vi "Basic Interface.vi"() -> ()   [LabVIEW 2019]
uses:
  source code/LSL components/scripts/scripts manager/scripts manager.lvclass
  source code/LSL components/output terminal/Plain OT/PainOutputTerminal.lvclass
  D:/Pet Projects/LSL/source code/LSL components/output terminal/Base/Output Terminal.lvclass
  source code/LSL components/output terminal/Plain OT/PainOutputTerminal.lvclass/PainOutputTerminal.ctl
  source code/LSL components/variables/RT Variables/RT Variables.lvclass
  source code/LSL components/scripts/scripts manager/scripts manager.lvclass/scripts manager.ctl
  source code/LSL components/output terminal/Plain OT/properties/Write Output Terminal.vi
  source code/LSL components/scripts/scripts manager/properties/Write Scripts.vi
panel:
  in  "Help":bool
  in  "Script Compile":bool
  in  "Script Save":bool
  in  "Script Delete":bool
  in  "Script New":bool
  in  "Script Run":bool
  in  "Script Files":i32(listbox)
  out "Output Terminal":string
  in  "scripting pane":T1
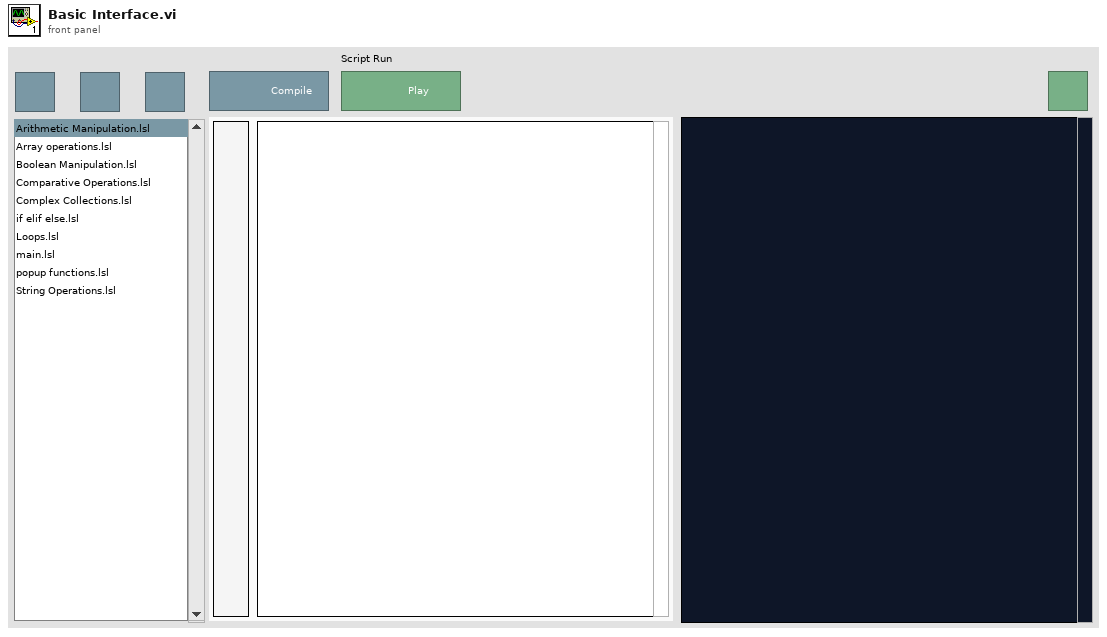
[diagram p1: front panel]
types:
  T1 = cluster{"Script Editor":string, "Script Editor":string}
  T2 = enum32{"Invalid", "Standard", "Closed", "Hidden", "Minimized", "Maximized"}
  T3 = enum32{"invalid app kind", "Development System", "Run Time System", "Student Edition", "Embedded LabVIEW", "Evaluation", "Custom"}
  T4 = cluster{"Core":cluster{"Current VI Reference":refnum<vi>, "Close Panel on Exit?":bool}, "scripts manager":refnum<class "scripts manager.lvclass">, "Script":string, "Config Folder":path, "PainOT":refnum<class "PainOutputTerminal.lvclass">}
  T5 = cluster{"Current VI Reference":refnum<vi>, "Close Panel on Exit?":bool}
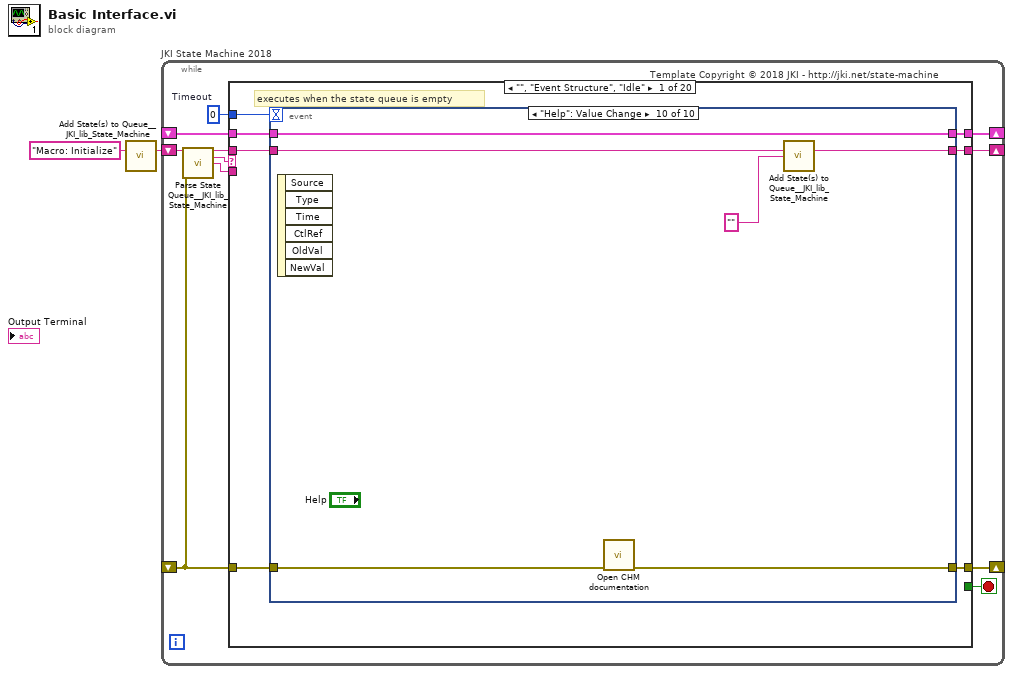
[diagram p0: block diagram]
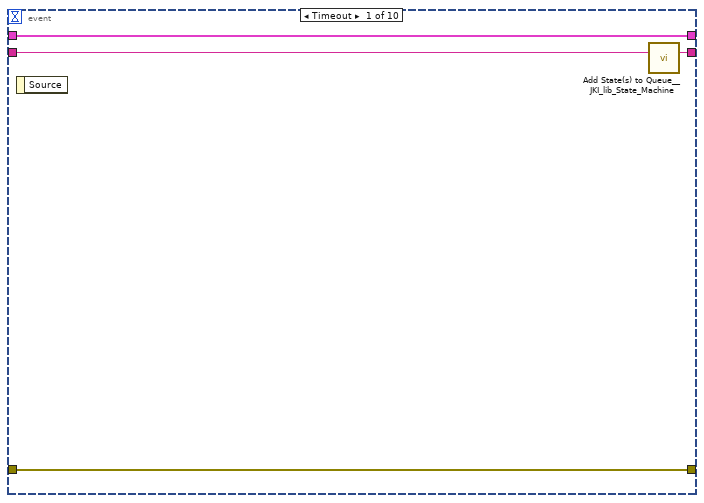
[diagram p2: hidden frame]
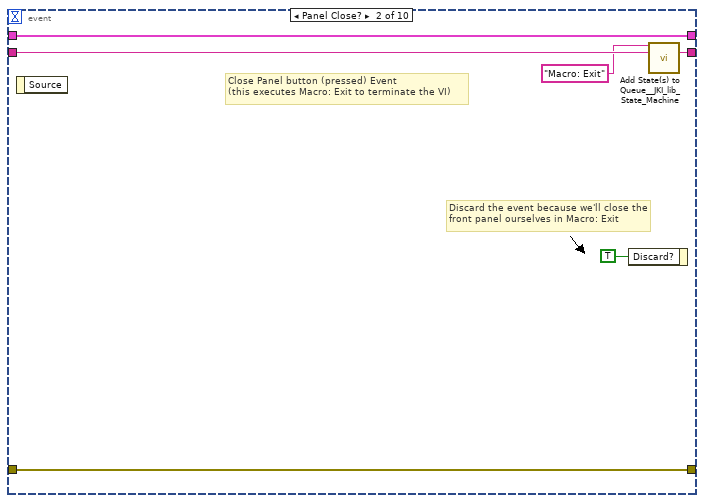
[diagram p3: hidden frame]
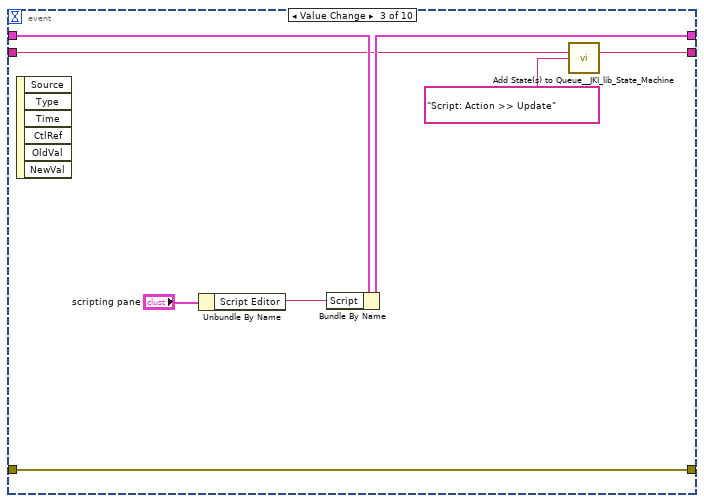
[diagram p4: hidden frame]
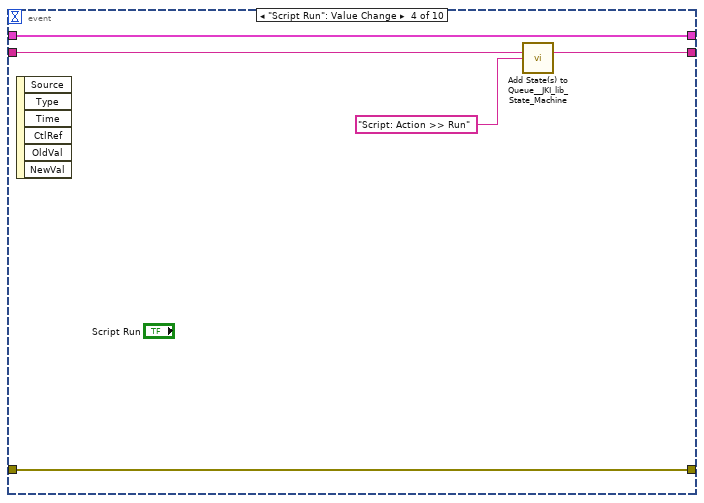
[diagram p5: hidden frame]
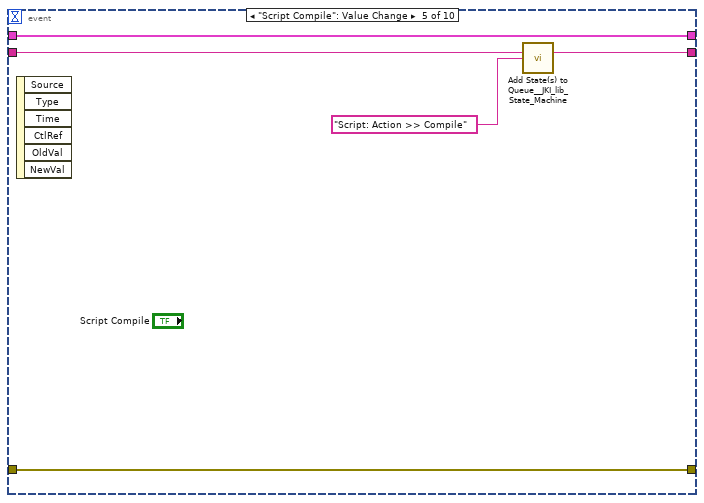
[diagram p6: hidden frame]
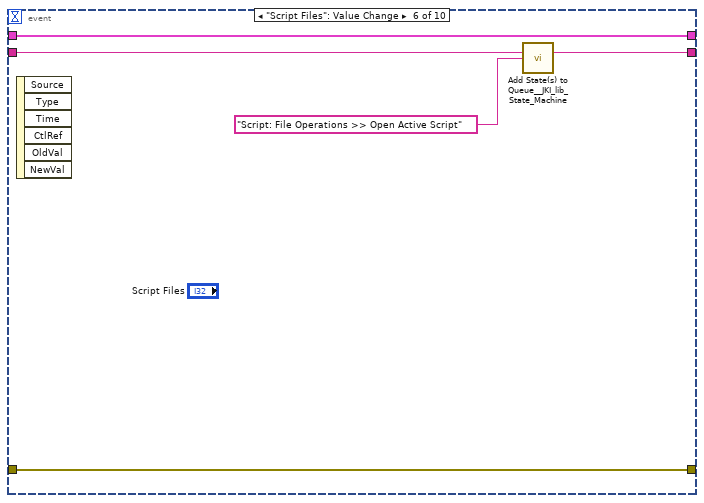
[diagram p7: hidden frame]
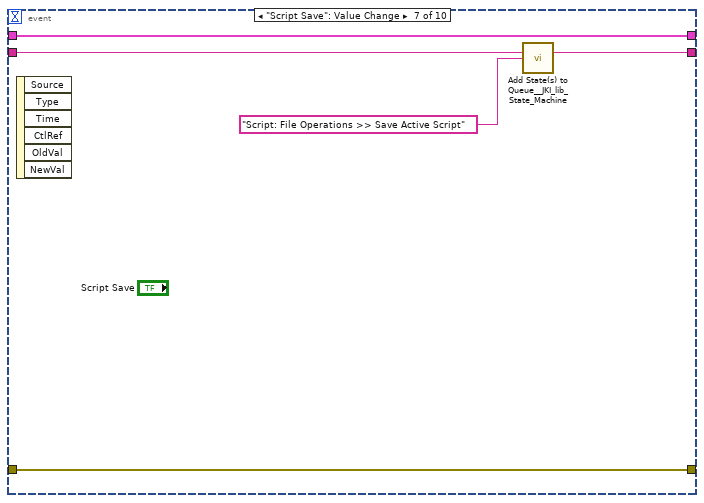
[diagram p8: hidden frame]
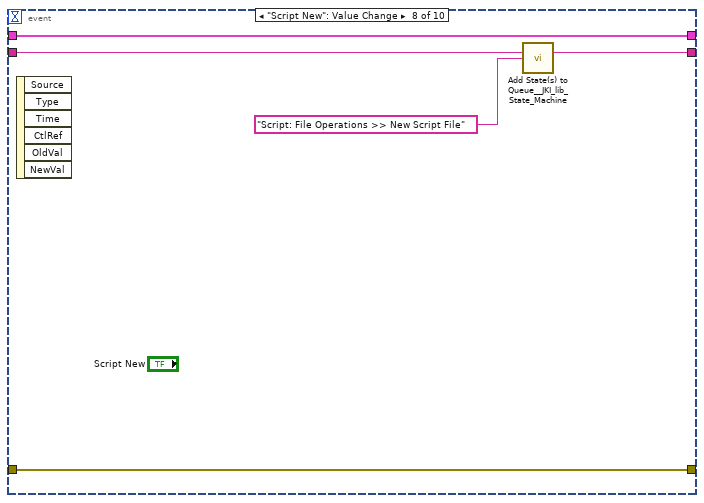
[diagram p9: hidden frame]
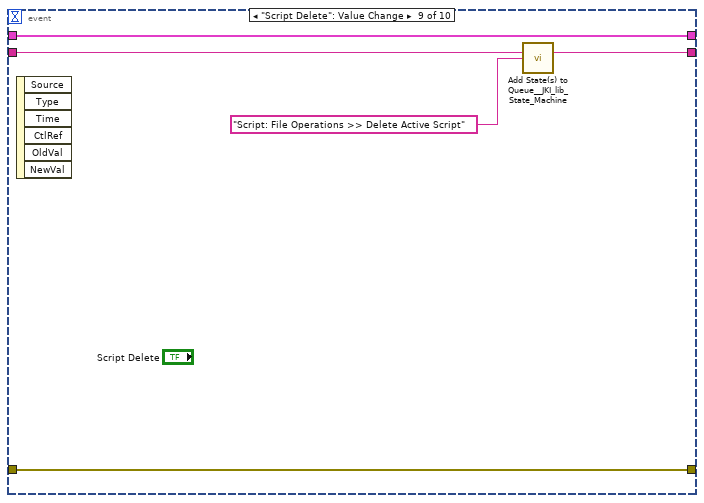
[diagram p10: hidden frame]
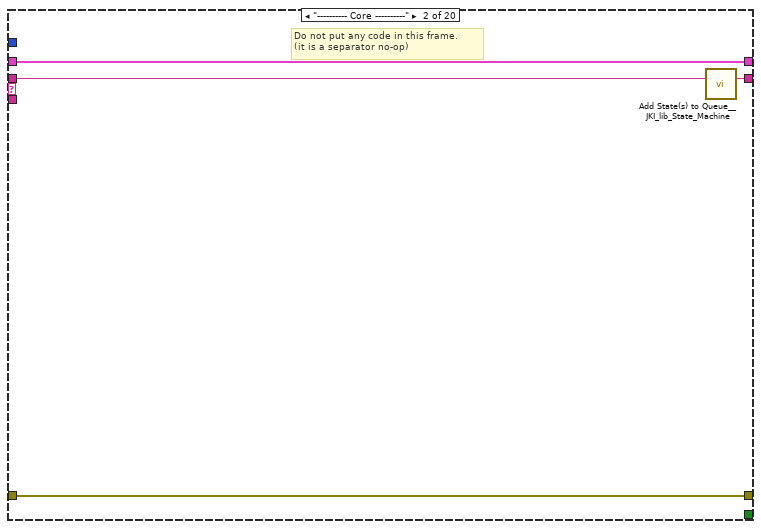
[diagram p11: hidden frame]
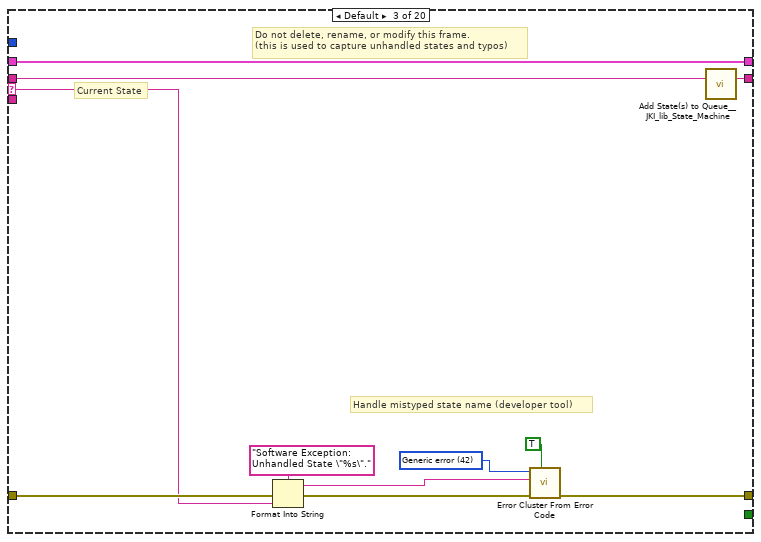
[diagram p12: hidden frame]
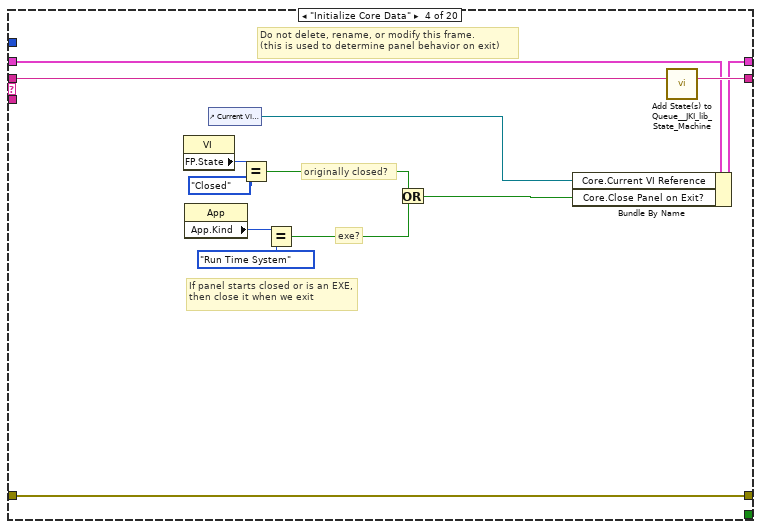
[diagram p13: hidden frame]
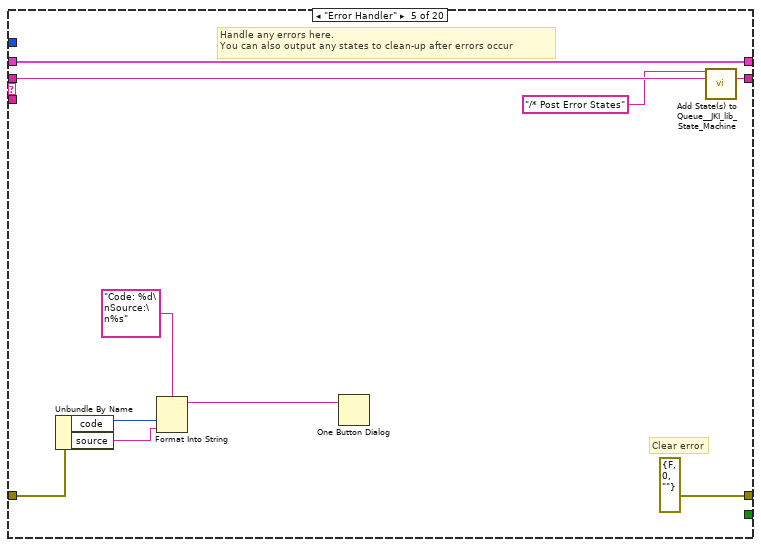
[diagram p14: hidden frame]
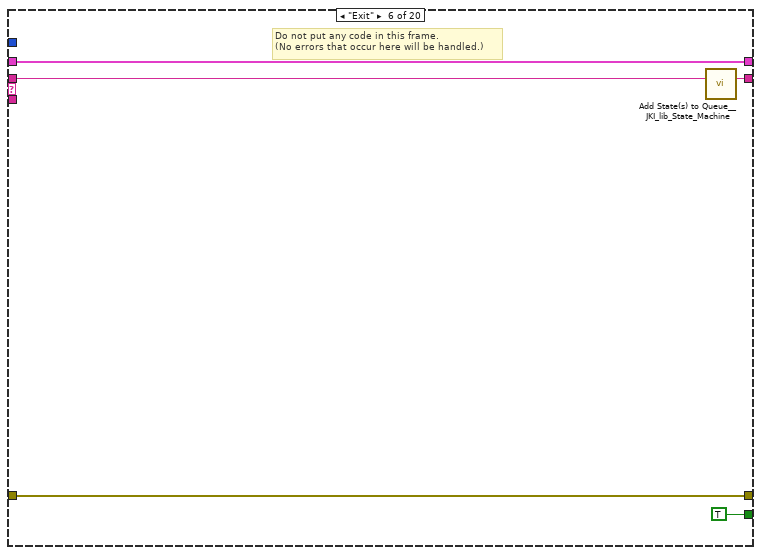
[diagram p15: hidden frame]
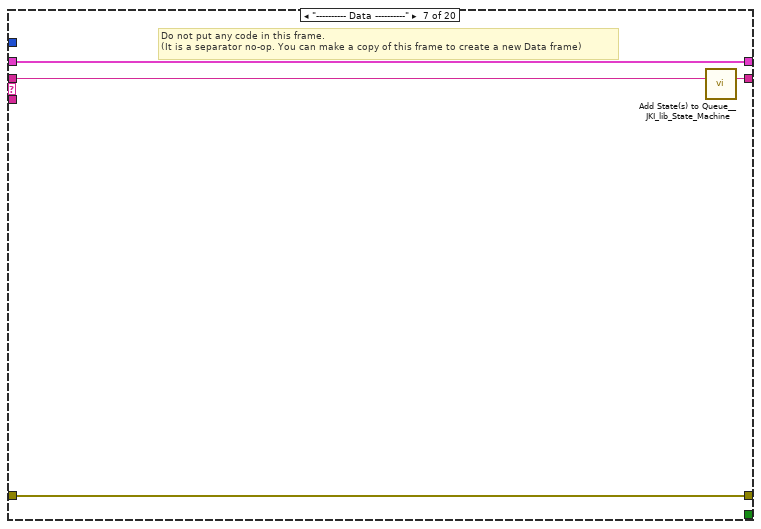
[diagram p16: hidden frame]
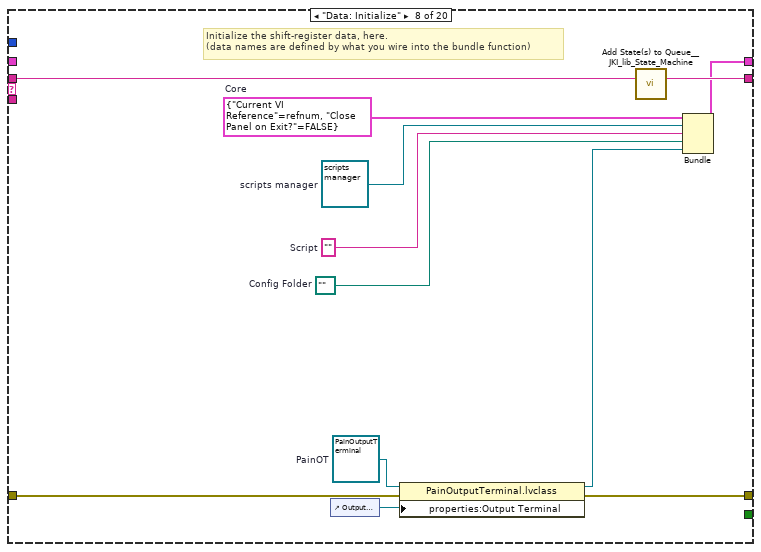
[diagram p17: hidden frame]
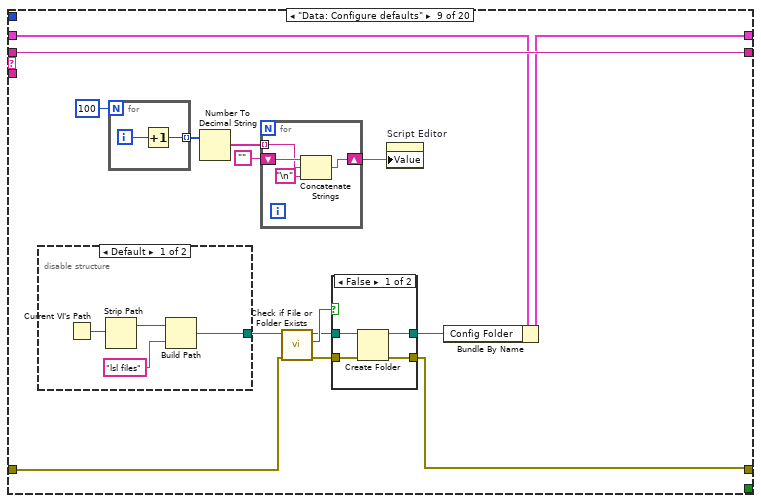
[diagram p18: hidden frame]
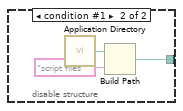
[diagram p19: hidden frame]
diagram:
  n1 = call <vilib>:"Add State(s) to Queue__JKI_lib_State_Machine.vi"("State(s) in (\"\")"="Macro: Initialize") -> ("States Out"=w2:string)  [unwired: 14 in]
  n2 = while "JKI State Machine 2018" {
    shift-right: [w6] -> _
    shift-left: _ -> [w5]
    shift-right: [w9] -> _
    shift-left: _ -> [w3]
    shift-right: [w8] -> _
    shift-left: w2 -> [w10]
    stop <- w7 stop-if-true
    w4 = 0  # Timeout
    # "Template Copyright © 2018 JKI - http://jki.net/state-machine"
    n3 = call <vilib>:"Parse State Queue__JKI_lib_State_Machine.vi"("State Queue"=w10, "Error In (no error)"=w3) -> ("Remaining States"=w12:string, "Current State"=w13:string, "Arguments"=w11:string)  [unwired: 11 in]
    n4 = case shown="\"\", \"Event Structure\", \"Idle\"" w13 {
      selector: w13 -> [_ _ w79 _ _ _ _ _ _ _ _ _ _ _ _ _ _ _ _ _]
      tunnel: w12 -> [w20 w78 w83 w102 w112 w117 w121 w133 w148 w173 w177 w189 w195 w206 w275 w280 w290 w294 w305 w335]
      tunnel: w11 -> [_ _ _ _ _ _ _ _ _ _ _ _ w190 w200 _ _ _ _ w303 w343]
      tunnel: w5 -> [w18 w75 w81 w95 w109 w115 w118 _ w141 w168 w174 w187 w193 w202 w272 w277 w287 w291 w298 w342]
      tunnel: [w17 w76 w85 w99 errorcluster {"status"=FALSE, "code"=0, "source"=""} ("error out") w114 w119 w124 w143 w169 w175 w184 w191 w203 w273 w278 w288 w292 w301 w344] -> w9
      tunnel: w3 -> [w16 w76 w84 w99 w107 w114 w119 w125 w144 w170 w175 w185 w192 w204 w273 w278 w288 w292 w302 w339]
      tunnel: [w19 w77 w82 w101 w111 w116 w120 w132 w148 w172 w176 w188 w194 w205 w274 w279 w289 w293 w304 w336] -> w8
      tunnel: [_ _ _ _ _ TRUE _ _ _ _ _ _ _ _ _ _ _ _ _ _] -> w7
      tunnel: [w15 w75 w81 w100 w109 w115 w118 w130 w140 w168 w174 w187 w193 w202 w272 w277 w287 w291 w297 w342] -> w6
      tunnel: w4 -> [w14 _ _ _ _ _ _ _ _ _ _ _ _ _ _ _ _ _ _ _]
      frame "", "Event Structure", "Idle" {
        # "executes when the state queue is empty"
        n5 = event shown="[9] \"Help\": Value Change" {
          selector: _ -> [_ _ _ _ _ _ _ _ _ _]
          dyn-events: _ -> [_ _ _ _ _ _ _ _ _ _]
          timeout: w14 -> [_ _ _ _ _ _ _ _ _ _]
          tunnel: w20 -> [w24 w30 w33 w40 w45 w50 w55 w60 w65 w72]
          tunnel: [w23 w29 w34 w41 w46 w51 w56 w61 w66 w73] -> w19
          tunnel: w18 -> [w21 w27 w36 w43 w48 w53 w58 w63 w68 w74]
          tunnel: [w22 w28 w31 w42 w47 w52 w57 w62 w67 w69] -> w17
          tunnel: w16 -> [w22 w28 w31 w42 w47 w52 w57 w62 w67 w70]
          tunnel: [w21 w27 w35 w43 w48 w53 w58 w63 w68 w74] -> w15
          event Timeout {
            n6 = event-data() -> ()  [unwired: 1 in, 1 out]
            n7 = call <vilib>:"Add State(s) to Queue__JKI_lib_State_Machine.vi"("State(s) in (\"\")"=w24) -> ("States Out"=w23:string)  [unwired: 14 in]
          }
          event Panel Close? {
            # "Discard the event because we'll close the front panel ourselves in Macro: Exit"
            # "Close Panel button (pressed) Event\n(this executes Macro: Exit to terminate the VI)"
            n8 = event-data() -> ()  [unwired: 1 in, 1 out]
            n9 = event-data("Discard?"=TRUE) -> ()  [unwired: 1 in, 1 out]
            n10 = call <vilib>:"Add State(s) to Queue__JKI_lib_State_Machine.vi"("State(s) in Front (\"\")"="Macro: Exit", "State(s) in (\"\")"=w30) -> ("States Out"=w29:string)  [unwired: 13 in]
          }
          event "scripting pane.Script Editor": Value Change {
            n11 = event-data() -> ()  [unwired: 1 in, 6 out]
            n12 = Unbundle By Name("scripting pane") -> ("Script Editor"=w37:string)
            n13 = Bundle By Name(cluster=w36, "Script"=w37) -> (w35:T4)
            n14 = call <vilib>:"Add State(s) to Queue__JKI_lib_State_Machine.vi"("State(s) in (\"\")"=w33, "State(s) at Back (\"\")"="Script: Action >> Update" ("State(s) at Back (\"\")")) -> ("States Out"=w34:string)  [unwired: 13 in]
          }
          event "Script Run": Value Change {
            n15 = event-data() -> ()  [unwired: 1 in, 6 out]
            n16 = call <vilib>:"Add State(s) to Queue__JKI_lib_State_Machine.vi"("State(s) in (\"\")"=w40, "State(s) at Back (\"\")"="Script: Action >> Run" ("State(s) at Back (\"\")")) -> ("States Out"=w41:string)  [unwired: 13 in]
          }
          event "Script Compile": Value Change {
            n17 = event-data() -> ()  [unwired: 1 in, 6 out]
            n18 = call <vilib>:"Add State(s) to Queue__JKI_lib_State_Machine.vi"("State(s) in (\"\")"=w45, "State(s) at Back (\"\")"="Script: Action >> Compile" ("State(s) at Back (\"\")")) -> ("States Out"=w46:string)  [unwired: 13 in]
          }
          event "Script Files": Value Change {
            n19 = event-data() -> ()  [unwired: 1 in, 6 out]
            n20 = call <vilib>:"Add State(s) to Queue__JKI_lib_State_Machine.vi"("State(s) in (\"\")"=w50, "State(s) at Back (\"\")"="Script: File Operations >> Open Active Script" ("State(s) at Back (\"\")")) -> ("States Out"=w51:string)  [unwired: 13 in]
          }
          event "Script Save": Value Change {
            n21 = event-data() -> ()  [unwired: 1 in, 6 out]
            n22 = call <vilib>:"Add State(s) to Queue__JKI_lib_State_Machine.vi"("State(s) in (\"\")"=w55, "State(s) at Back (\"\")"="Script: File Operations >> Save Active Script" ("State(s) at Back (\"\")")) -> ("States Out"=w56:string)  [unwired: 13 in]
          }
          event "Script New": Value Change {
            n23 = event-data() -> ()  [unwired: 1 in, 6 out]
            n24 = call <vilib>:"Add State(s) to Queue__JKI_lib_State_Machine.vi"("State(s) in (\"\")"=w60, "State(s) at Back (\"\")"="Script: File Operations >> New Script File" ("State(s) at Back (\"\")")) -> ("States Out"=w61:string)  [unwired: 13 in]
          }
          event "Script Delete": Value Change {
            n25 = event-data() -> ()  [unwired: 1 in, 6 out]
            n26 = call <vilib>:"Add State(s) to Queue__JKI_lib_State_Machine.vi"("State(s) in (\"\")"=w65, "State(s) at Back (\"\")"="Script: File Operations >> Delete Active Script" ("State(s) at Back (\"\")")) -> ("States Out"=w66:string)  [unwired: 13 in]
          }
          event "Help": Value Change {
            n27 = event-data() -> ()  [unwired: 1 in, 6 out]
            n28 = call "Open CHM documentation.vi"("error in"=w70) -> ("error out"=w69:errorcluster)  [unwired: 10 in]
            n29 = call <vilib>:"Add State(s) to Queue__JKI_lib_State_Machine.vi"("State(s) in (\"\")"=w72, "State(s) at Back (\"\")"="" ("State(s) at Back (\"\")")) -> ("States Out"=w73:string)  [unwired: 13 in]
          }
        }
      }
      frame "---------- Core ----------" {
        # "Do not put any code in this frame.\n(it is a separator no-op)"
        n30 = call <vilib>:"Add State(s) to Queue__JKI_lib_State_Machine.vi"("State(s) in (\"\")"=w78) -> ("States Out"=w77:string)  [unwired: 14 in]
      }
      frame Default {
        w88 = 42 items=["No error", "Argument error", "Memory is full", "Out of zone", "End of file", "File already open", "Generic file I/O error", "File not found", "File permission error", "Disk is full", "Duplicate path", "Too many files open", "System feature not enabled", "Resource file not found", "Cannot add resource", "Resource not found", "Image not found", "Image memory error", "Pen does not exist", "Config type invalid", "Config token not found", "Config parse error", "Config memory error", "Bad external code format", "Bad external code offset", "External code not present", "Null window", "Destroy window error", "Null menu", "Print aborted", "Bad print record", "Print driver error", "Windows error during printing", "Memory error during printing", "Print dialog error", "Generic print error", "Invalid device refnum", "Device not found", "Device parameter error", "Device unit error", "Cannot open device", "Device call aborted", "Generic error", "Cancelled by user", "Object ID too low", "Object ID too high", "Object not in heap", "Unknown heap", "Unknown object (invalid DefProc)", "Unknown object (DefProc not in table)", "Message out of range", "Invalid (null) method", "Unknown message", "Manager call not supported", "Bad address", "Network operation in progress", "Network operation timed out", "Connection is busy", "Network attribute not supported", "Network error", "Address in use", "System out of memory", "Connection aborted", "Connection refused", "Not connected", "Already connected", "Connection closed", "Initialization error (interapplication manager)", "Bad occurrence", "Wait on unbound occurrence handler", "Occurrence queue overflow", "Datalog type conflict", "Unused", "Unrecognized type (interapplication manager)", "Memory corrupt", "Failed to make temporary DLL", "Old CIN version", "Drag socket not found", "Failed to load drop-object", "Failed to register OLE object", "Failed to release OLE object", "Format specifier type mismatch", "Unknown format specifier", "Too few format specifiers", "Too many format specifiers", "Scan failed", "Newer CIN version", "Error converting to variant", "Runtime menu error", "Password tampered", "Variant attribute not found", "Incompatible variant data type", "Event data is not available", "Event Store is not present", "Occurrence is not found", "Event Queue is not created", "Event info is not available", "Refnum passed is NULL", "Error retrieving Class GUID", "Error retrieving CoClass GUID", "Error retrieving TypeLib GUID.", "Bad built application magic bytes.", "Specific driver is different from the specific driver associated with the Logical Name.", "There is no session opened to the class driver.", "Max Error", "MAX - Error with config objects", "MAX - Error loading configuration", "MAX - Group not supported"]
        # "Current State"
        # "Do not delete, rename, or modify this frame.\n(this is used to capture unhandled states and typos)"
        # "Handle mistyped state name (developer tool)"
        n31 = Format Into String(format string="Software Exception: Unhandled State \"%s\"." ("message"), error in=w84, w79) -> (resulting string=w87:string, error out=w86:errorcluster)  [unwired: 1 in]
        n32 = call <vilib>:"Error Cluster From Error Code.vi"("show call chain? (False)"=TRUE, "error in (no error)"=w86, "error message (\"\")"=w87, "error code (0)"=w88) -> ("error out"=w85:errorcluster)  [unwired: 5 in]
        n33 = call <vilib>:"Add State(s) to Queue__JKI_lib_State_Machine.vi"("State(s) in (\"\")"=w83) -> ("States Out"=w82:string)  [unwired: 14 in]
      }
      frame "Initialize Core Data" {
        # "Do not delete, rename, or modify this frame.\n(this is used to determine panel behavior on exit)"
        # "originally closed?"
        # "exe?"
        # "If panel starts closed or is an EXE, then close it when we exit"
        n34 = property class="VI"() -> ("FP.State"=w92:T2)  [unwired: 2 in, 2 out]
        n35 = property class="App"() -> ("App.Kind"=w98:T3)  [unwired: 2 in, 2 out]
        n36 = control-ref of="Current VI Reference"() -> (w93:refnum<vi>)
        n37 = Equal?(x=w92, y=T2."Closed" ("Front Panel Window:State")) -> (x = y?=w90:bool)
        n38 = Equal?(x=w98, y=T3."Run Time System" ("Application:Kind")) -> (x = y?=w96:bool)
        n39 = Or(x=w90, y=w96) -> (x .or. y?=w94:bool)
        n40 = Bundle By Name(cluster=w95, "Core.Current VI Reference"=w93, "Core.Close Panel on Exit?"=w94) -> (w100:T4)
        n41 = call <vilib>:"Add State(s) to Queue__JKI_lib_State_Machine.vi"("State(s) in (\"\")"=w102) -> ("States Out"=w101:string)  [unwired: 14 in]
      }
      frame "Error Handler" {
        # "Handle any errors here.\nYou can also output any states to clean-up after errors occur"
        # "Clear error"
        n42 = Unbundle By Name(w107) -> ("code"=w106:i32, "source"=w105:string)
        n43 = Format Into String(format string="Code: %d\nSource:\n%s", w106, w105) -> (resulting string=w103:string)  [unwired: 2 in, 1 out]
        n44 = One Button Dialog(message=w103) -> ()  [unwired: 1 in, 1 out]
        n45 = call <vilib>:"Add State(s) to Queue__JKI_lib_State_Machine.vi"("State(s) in Front (\"\")"="/* Post Error States", "State(s) in (\"\")"=w112) -> ("States Out"=w111:string)  [unwired: 13 in]
      }
      frame "Exit" {
        # "Do not put any code in this frame.\n(No errors that occur here will be handled.)"
        n46 = call <vilib>:"Add State(s) to Queue__JKI_lib_State_Machine.vi"("State(s) in (\"\")"=w117) -> ("States Out"=w116:string)  [unwired: 14 in]
      }
      frame "---------- Data ----------" {
        # "Do not put any code in this frame.\n(It is a separator no-op. You can make a copy of this frame to create a new Data frame)"
        n47 = call <vilib>:"Add State(s) to Queue__JKI_lib_State_Machine.vi"("State(s) in (\"\")"=w121) -> ("States Out"=w120:string)  [unwired: 14 in]
      }
      frame "Data: Initialize" {
        w122 = path ""  # Config Folder
        w127 = refnum<class "PainOutputTerminal.lvclass"> refnum  # PainOT
        w128 = ""  # Script
        w129 = refnum<class "scripts manager.lvclass"> refnum  # scripts manager
        w131 = T5 {"Current VI Reference"=refnum, "Close Panel on Exit?"=FALSE}  # Core
        # "Initialize the shift-register data, here.\n(data names are defined by what you wire into the bundle function)"
        n48 = control-ref of="Output Terminal"() -> (w123:refnum<vi>)
        n49 = property class="PainOutputTerminal.lvclass"(reference=w127, error in=w125, "properties:Output Terminal"=w123) -> (reference out=w126:refnum<class "PainOutputTerminal.lvclass">, error out=w124:errorcluster)
        n50 = call <vilib>:"Add State(s) to Queue__JKI_lib_State_Machine.vi"("State(s) in (\"\")"=w133) -> ("States Out"=w132:string)  [unwired: 14 in]
        n51 = Bundle("Core"=w131, "scripts manager"=w129, "Script"=w128, "Config Folder"=w122, "PainOT"=w126) -> (w130:T4)  [unwired: 1 in]
      }
      frame "Data: Configure defaults" {
        n52 = disable-structure shown="Default" {
          disable-tunnel: [w149 w153] -> w134
          frame condition #0 (active) {
            n53 = Current VI's Path() -> (path=w152:path)
            n54 = Strip Path(path=w152) -> (stripped path=w151:path)  [unwired: 1 out]
            n55 = Build Path(base path=w151, name or relative path="lsl files") -> (appended path=w149:path)
          }
          frame condition #1 {
            n56 = call <vilib>:"Application Directory.vi"() -> ("Application Directory"=w154:path)
            n57 = Build Path(base path=w154, name or relative path="script files") -> (appended path=w153:path)
          }
        }
        n58 = for {
          N: 100 -> [_]
          tunnel: [w160] -> w138 mode=indexing
          i -> [w161]
          n59 = Increment(x=w161) -> (x+1=w160:i32)
        }
        n60 = Number To Decimal String(number=w138) -> (decimal integer string=w136:string[])  [unwired: 1 in]
        n61 = for {
          tunnel: w136 -> [w156] mode=indexing
          shift-right: [w159] -> w137
          shift-left: "" -> [w157]
          n62 = Concatenate Strings(w157, w156, "\n") -> (w159:string)
        }
        n63 = call <vilib>:"Check if File or Folder Exists.vi"("error in (no error)"=w144, "path"=w134) -> ("error out"=w145:errorcluster, "file or folder exists?"=w147:bool, "dup path"=w146:path)  [unwired: 7 in]
        n64 = case shown="False" w147 {
          tunnel: w145 -> [w165 w166]
          tunnel: w146 -> [w164 w167]
          tunnel: [w162 w167] -> w142
          tunnel: [w163 w166] -> w143
          frame False {
            n65 = Create Folder(path (use dialog)=w164, error in=w165) -> (created path=w162:path, error out=w163:errorcluster)  [unwired: 1 in, 1 out]
          }
          frame True {
          }
        }
        n66 = property on="Script Editor" class="Str"("Value"=w137) -> ()  [unwired: 2 in, 2 out]
        n67 = Bundle By Name(cluster=w141, "Config Folder"=w142) -> (w140:T4)
      }
      frame "Data: Cleanup" {
        # "Cleanup any data and references, here.\n(this is called automatically, by the Macro: Exit)"
        n68 = Unbundle By Name(w168) -> ("Core.Current VI Reference"=w171:refnum<vi>)
        n69 = Close Reference(reference=w171, error in (no error)=w170) -> (error out=w169:errorcluster)
        n70 = call <vilib>:"Add State(s) to Queue__JKI_lib_State_Machine.vi"("State(s) in (\"\")"=w173) -> ("States Out"=w172:string)  [unwired: 14 in]
      }
      frame "---------- UI ----------" {
        # "Do not put any code in this frame.\n(It is a separator no-op. You can make a copy of this frame to create a new UI frame)"
        n71 = call <vilib>:"Add State(s) to Queue__JKI_lib_State_Machine.vi"("State(s) in (\"\")"=w177) -> ("States Out"=w176:string)  [unwired: 14 in]
      }
      frame "UI: Initialize" {
        w182 = u32 923176
        # "Initialize the User Interface, here.\n(this is called automatically, by the Macro: Init)"
        n72 = property on="Script Editor" class="Str"("Text.BG Color"=u32 16119285) -> ()  [unwired: 2 in, 2 out]
        n73 = property on="Output Terminal" class="Str"("Text.BG Color"=w182, "Text.BGColor"=w182, "Text.TextColor"=u32 16777215) -> ()  [unwired: 2 in, 2 out]
        n74 = property on="Script Files" class="LstBox (strict)"("Item Names"=string[] []) -> ()  [unwired: 2 in, 2 out]
        n75 = property on="Script Files" class="LstBox (strict)"(error in=w185, "SelColor"=u32 8034469) -> (error out=w184:errorcluster)  [unwired: 1 in, 1 out]
        n76 = local write "Output Terminal"("" ("Output Terminal")) -> ()
        n77 = local write "scripting pane"(T1 {"Script Editor"="", "Script Editor"=""} ("scripting pane")) -> ()
        n78 = call <vilib>:"Add State(s) to Queue__JKI_lib_State_Machine.vi"("State(s) in (\"\")"=w189) -> ("States Out"=w188:string)  [unwired: 14 in]
      }
      frame "UI: Cursor Set" {
        # "Argument"
        # "Set and Unset Cursor Busy.\n(Usage: \"UI: Cursor Set >> Busy|Idle\")"
        n79 = case shown="\"Idle\", Default" w190 {
          tunnel: w192 -> [w197 w199]
          tunnel: [w196 w198] -> w191
          frame "Idle", Default {
            n80 = call <vilib>:"Unset Busy.vi"("error in (no error)"=w197) -> ("error out"=w196:errorcluster)  [unwired: 10 in]
          }
          frame "Busy" {
            n81 = call <vilib>:"Set Busy.vi"("error in (no error)"=w199) -> ("error out"=w198:errorcluster)  [unwired: 9 in, 1 out]
          }
        }
        n82 = call <vilib>:"Add State(s) to Queue__JKI_lib_State_Machine.vi"("State(s) in (\"\")"=w195) -> ("States Out"=w194:string)  [unwired: 14 in]
      }
      frame "UI: Front Panel State" {
        # "Argument"
        # "Set Front Panel Open or Closed\n(Usage: \"UI: Front Panel State >> Open|Close\")"
        n83 = Unbundle By Name(w202) -> ("Core.Current VI Reference"=w201:refnum<vi>)
        n84 = case shown="\"Maximize\", \"Maximized\"" w200 {
          tunnel: w204 -> [w212 w227 w238 w251 w264]
          tunnel: [w214 w228 w240 w253 w266] -> w203
          tunnel: w201 -> [w213 w225 w239 w252 w265]
          frame "Open", "Standard", Default {
            w207 = T2."Standard" ("State")
            n85 = property class="VI"(reference=w213, error in=w212) -> (reference out=w210:refnum<vi>, error out=w211:errorcluster, "FP.State"=w209:T2)
            n86 = Not Equal?(x=w209, y=w207) -> (x != y?=w208:bool)
            n87 = case shown="True" w208 {
              tunnel: [w218 w220] -> w214
              tunnel: w211 -> [w217 w220]
              tunnel: w210 -> [w216 _]
              tunnel: w207 -> [w215 _]
              frame True {
                n88 = invoke class="VI" method="FP.Open"(reference=w216, error in=w217, "Activate"=TRUE, "State"=w215) -> (error out=w218:errorcluster)  [unwired: 1 in, 4 out]
              }
              frame False {
              }
            }
          }
          frame "Close", "Closed" {
            n89 = property class="VI"(reference=w225, error in=w227) -> (reference out=w224:refnum<vi>, error out=w226:errorcluster, "FP.State"=w222:T2)
            n90 = Not Equal?(x=w222, y=T2."Closed" ("Front Panel Window:State")) -> (x != y?=w221:bool)
            n91 = case shown="True" w221 {
              tunnel: [w229 w232] -> w228
              tunnel: w226 -> [w229 w231]
              tunnel: w224 -> [_ w230]
              frame False {
              }
              frame True {
                n92 = invoke class="VI" method="FP.Close"(reference=w230, error in=w231) -> (error out=w232:errorcluster)  [unwired: 1 in, 2 out]
              }
            }
          }
          frame "Hidden", "Hide" {
            w233 = T2."Hidden" ("State")
            n93 = property class="VI"(reference=w239, error in=w238) -> (reference out=w236:refnum<vi>, error out=w237:errorcluster, "FP.State"=w235:T2)
            n94 = Not Equal?(x=w235, y=w233) -> (x != y?=w234:bool)
            n95 = case shown="True" w234 {
              tunnel: [w244 w245] -> w240
              tunnel: w237 -> [w243 w245]
              tunnel: w236 -> [w242 _]
              tunnel: w233 -> [w241 _]
              frame True {
                n96 = invoke class="VI" method="FP.Open"(reference=w242, error in=w243, "State"=w241) -> (error out=w244:errorcluster)  [unwired: 2 in, 4 out]
              }
              frame False {
              }
            }
          }
          frame "Minimize", "Minimized" {
            w246 = T2."Minimized" ("State")
            n97 = property class="VI"(reference=w252, error in=w251) -> (reference out=w249:refnum<vi>, error out=w250:errorcluster, "FP.State"=w248:T2)
            n98 = Not Equal?(x=w248, y=w246) -> (x != y?=w247:bool)
            n99 = case shown="True" w247 {
              tunnel: [w257 w258] -> w253
              tunnel: w250 -> [w256 w258]
              tunnel: w249 -> [w255 _]
              tunnel: w246 -> [w254 _]
              frame True {
                n100 = invoke class="VI" method="FP.Open"(reference=w255, error in=w256, "State"=w254) -> (error out=w257:errorcluster)  [unwired: 2 in, 4 out]
              }
              frame False {
              }
            }
          }
          frame "Maximize", "Maximized" {
            w259 = T2."Maximized" ("State")
            n101 = property class="VI"(reference=w265, error in=w264) -> (reference out=w262:refnum<vi>, error out=w263:errorcluster, "FP.State"=w261:T2)
            n102 = Not Equal?(x=w261, y=w259) -> (x != y?=w260:bool)
            n103 = case shown="True" w260 {
              tunnel: [w270 w271] -> w266
              tunnel: w263 -> [w269 w271]
              tunnel: w262 -> [w268 _]
              tunnel: w259 -> [w267 _]
              frame True {
                n104 = invoke class="VI" method="FP.Open"(reference=w268, error in=w269, "State"=w267) -> (error out=w270:errorcluster)  [unwired: 2 in, 4 out]
              }
              frame False {
              }
            }
          }
        }
        n105 = call <vilib>:"Add State(s) to Queue__JKI_lib_State_Machine.vi"("State(s) in (\"\")"=w206) -> ("States Out"=w205:string)  [unwired: 14 in]
      }
      frame "---------- Macro ----------" {
        # "Do not put any code in this frame.\n(It is a separator no-op. You can make a copy of this frame to create a new Macro frame)"
        n106 = call <vilib>:"Add State(s) to Queue__JKI_lib_State_Machine.vi"("State(s) in (\"\")"=w275) -> ("States Out"=w274:string)  [unwired: 14 in]
      }
      frame "Macro: Initialize" {
        w276 = "Data: Initialize\nInitialize Core Data\nUI: Initialize\nUI: Front Panel State >> Open\nData: Configure defaults\n\nScript: Action >> Init\nScript: File Operations >>List Script File\nScript: File Operations >> Open Active Script"  # Data: Initialize Initialize Core Data UI: Initialize UI: Front Panel State >> Open Data: Configure defaults  Script: Action >> Init Script: File Operations >>List Script File Script: File Operations >> Open Active Script
        # "Initialization Macro\n(This is called once, when the VI starts)"
        n107 = call <vilib>:"Add State(s) to Queue__JKI_lib_State_Machine.vi"("State(s) in Front (\"\")"=w276, "State(s) in (\"\")"=w280) -> ("States Out"=w279:string)  [unwired: 13 in]
      }
      frame "Macro: Exit" {
        # "Exit Macro\n(This is called once, when the VI exits)"
        n108 = Unbundle By Name(w287) -> ("Core.Close Panel on Exit?"=w286:bool)
        n109 = Select(t="UI: Front Panel State >> Close", s=w286, f="") -> (s? t:f=w283:string)
        n110 = call <vilib>:"Add State(s) to Queue__JKI_lib_State_Machine.vi"("State(s) in (\"\")"=w283, "State(s) at Back (\"\")"="Data: Cleanup\n\nScript: Action >> Close\n\nExit") -> ("States Out"=w281:string)  [unwired: 13 in]
        n111 = call <vilib>:"Add State(s) to Queue__JKI_lib_State_Machine.vi"("State(s) in Front (\"\")"=w281, "State(s) in (\"\")"=w290) -> ("States Out"=w289:string)  [unwired: 13 in]
      }
      frame "---------- Script ----------" {
        # "Template Separator\n(You can make a copy of, or modify, this frame)"
        n112 = call <vilib>:"Add State(s) to Queue__JKI_lib_State_Machine.vi"("State(s) in (\"\")"=w294) -> ("States Out"=w293:string)  [unwired: 14 in]
      }
      frame "Script: Action" {
        n113 = Unbundle By Name(w298) -> ("PainOT"=w295:refnum<class "PainOutputTerminal.lvclass">, "Script"=w296:string, "scripts manager"=w300:refnum<class "scripts manager.lvclass">)
        n114 = case shown="\"Init\"" w303 {
          tunnel: w302 -> [w306 w313 w318 w322 w328 w331]
          tunnel: [w306 w312 w316 w320 w324 w330] -> w301
          tunnel: w300 -> [w307 _ w317 w321 w327 w332]
          tunnel: [w307 w311 w315 w319 w323 refnum<class "scripts manager.lvclass"> refnum ("scripts manager out")] -> w299
          tunnel: w296 -> [_ _ w314 _ _ _]
          tunnel: w295 -> [_ w308 _ _ _ _]
          frame Default {
          }
          frame "Init" {
            w309 = refnum<class "RT Variables.lvclass"> refnum  # RT Variables
            w310 = refnum<class "scripts manager.lvclass"> refnum  # scripts manager
            n115 = call-dynamic "Instantiate.vi"("scripts manager in"=w310, "Output Terminal"=w308, "RT Variables"=w309, "error in (no error)"=w313) -> ("scripts manager out"=w311:refnum<class "scripts manager.lvclass">, "error out"=w312:errorcluster)  [unwired: 10 in]
          }
          frame "Update" {
            n116 = property class="scripts manager.lvclass"(reference=w317, error in=w318, "properties:Scripts"=w314) -> (reference out=w315:refnum<class "scripts manager.lvclass">, error out=w316:errorcluster)
          }
          frame "Compile" {
            n117 = call-dynamic "Compile Script.vi"("scripts manager in"=w321, "error in (no error)"=w322) -> ("scripts manager out"=w319:refnum<class "scripts manager.lvclass">, "error out"=w320:errorcluster)  [unwired: 12 in]
          }
          frame "Run" {
            n118 = call-dynamic "Compile Script.vi"("scripts manager in"=w327, "error in (no error)"=w328) -> ("scripts manager out"=w326:refnum<class "scripts manager.lvclass">, "error out"=w325:errorcluster)  [unwired: 12 in]
            n119 = call-dynamic "Execute Script.vi"("scripts manager in"=w326, "error in (no error)"=w325) -> ("scripts manager out"=w323:refnum<class "scripts manager.lvclass">, "error out"=w324:errorcluster)  [unwired: 12 in]
          }
          frame "Close" {
            n120 = call-dynamic "Destroy.vi"("scripts manager in"=w332, "error in (no error)"=w331) -> ("error out"=w330:errorcluster)  [unwired: 12 in, 1 out]
          }
        }
        n121 = Bundle By Name(cluster=w298, "scripts manager"=w299) -> (w297:T4)
        n122 = call <vilib>:"Add State(s) to Queue__JKI_lib_State_Machine.vi"("State(s) in (\"\")"=w305) -> ("States Out"=w304:string)  [unwired: 14 in]
      }
      frame "Script: File Operations" {
        n123 = property on="Script Files" class="LstBox (strict)"() -> ("Item Names"=w337:string[], "Value"=w333:i32)  [unwired: 2 in, 2 out]
        n124 = Unbundle By Name(w342) -> ("Config Folder"=w338:path, "Script"=w341:string)
        n125 = Index Array(array=w337, index=w333) -> (element=w340:string)
        n126 = case shown="\"List Script File\"" w343 {
          tunnel: w339 -> [w345 w355 w361 w368 w374 w397]
          tunnel: [w345 w352 w359 w366 w378 w392] -> w344
          tunnel: w341 -> [_ _ _ w365 _ _]
          tunnel: w340 -> [_ _ w357 w364 w376 _]
          tunnel: w338 -> [_ w346 w356 w363 w377 _]
          tunnel: w337 -> [_ _ _ _ w372 w393]
          tunnel: [_ _ _ _ w370 w389] -> w334
          tunnel: w333 -> [_ _ _ _ w371 _]
          frame Default {
          }
          frame "List Script File" {
            n127 = List Folder(path=w346, pattern="*.lsl", error in=w355) -> (filenames=w349:string[], error out=w353:errorcluster)  [unwired: 1 in, 2 out]
            n128 = Empty Array?(array=w349) -> (empty?=w350:bool)
            n129 = Select(t=string[] ["main.lsl"], s=w350, f=w349) -> (s? t:f=w348:string[])
            n130 = property on="Script Files" class="LstBox (strict)"(error in=w353, "Item Names"=w348, "Value"=0 ("Files")) -> (error out=w352:errorcluster)  [unwired: 1 in, 1 out]
          }
          frame "Open Active Script" {
            n131 = Build Path(base path=w356, name or relative path=w357) -> (appended path=w362:path)
            n132 = Read from Text File(file (use dialog)=w362, error in=w361) -> (text=w358:string, error out=w360:errorcluster)  [unwired: 2 in, 2 out]
            n133 = property on="Script Editor" class="Str"("Val(Sgnl)"=w358) -> ()  [unwired: 2 in, 2 out]
            n134 = call <vilib>:"Clear Errors.vi"("error in (no error)"=w360) -> ("error out"=w359:errorcluster)  [unwired: 5 in, 1 out]
          }
          frame "Save Active Script" {
            n135 = Build Path(base path=w363, name or relative path=w364) -> (appended path=w369:path)
            n136 = Write to Text File(file (use dialog)=w369, text=w365, error in=w368) -> (error out=w367:errorcluster)  [unwired: 1 in, 2 out]
            n137 = call <vilib>:"Clear Errors.vi"("error in (no error)"=w367) -> ("error out"=w366:errorcluster)  [unwired: 5 in, 1 out]
          }
          frame "Delete Active Script" {
            n138 = Build Path(base path=w377, name or relative path=w376) -> (appended path=w375:path)
            n139 = case shown="Default" w376 {
              tunnel: w375 -> [w386 _]
              tunnel: w374 -> [w387 w388]
              tunnel: [w385 w388] -> w373
              tunnel: w372 -> [w384 _]
              tunnel: w371 -> [w381 _]
              tunnel: ["Script: File Operations >> Open Active Script" _] -> w370
              frame Default {
                n140 = Delete From Array(array=w384, length=1, index=w381) -> (array with subset deleted=w383:string[])  [unwired: 1 out]
                n141 = Delete(path (use dialog)=w386, error in=w387) -> (error out=w385:errorcluster)  [unwired: 3 in, 2 out]
                n142 = property on="Script Files" class="LstBox (strict)"("Item Names"=w383, "Value"=0 ("Script Files")) -> ()  [unwired: 2 in, 2 out]
              }
              frame "main.lsl" {
              }
            }
            n143 = call <vilib>:"Clear Errors.vi"("error in (no error)"=w373) -> ("error out"=w378:errorcluster)  [unwired: 5 in, 1 out]
          }
          frame "New Script File" {
            n144 = call "New Script File"("error in (no error)"=w397) -> ("File Name"=w394:string, "Create"=w395:bool, "error out"=w396:errorcluster)  [unwired: 16 in]
            n145 = Concatenate Strings(w394, ".lsl" ("string")) -> (w391:string)
            n146 = case shown="True" w395 {
              tunnel: w396 -> [w398 w400]
              tunnel: w391 -> [_ w404]
              tunnel: w393 -> [_ w402]
              tunnel: [w398 w400] -> w392
              tunnel: [_ "Script: File Operations >> Open Active Script"] -> w389
              frame False {
              }
              frame True {
                n147 = Build Array (concatenate)(w402, w404) -> (w403:string[])
                n148 = Array Size(array=w402) -> (size(s)=w401:i32)
                n149 = property on="Script Files" class="LstBox (strict)"("Item Names"=w403, "Value"=w401) -> ()  [unwired: 2 in, 2 out]
              }
            }
          }
        }
        n150 = call <vilib>:"Add State(s) to Queue__jki_lib_state_machine.vi"("State(s) in Front (\"\")"=w334, "State(s) in (\"\")"=w335) -> ("States Out"=w336:string)  [unwired: 13 in]
      }
    }
  }
